vi "MessageHandlerProcess.vi"(10 "InitString":string, 11 "EVE reference in":refnum<data-value>) -> ()   [LabVIEW 2013]
uses:
  001 - MAIN/Class/EVE/EVE.lvclass
  Class/MessageHandler.lvclass
  030 - EVENTS/03 - ToMessageHandlerProcess/enumMessageCriticity.ctl
  030 - EVENTS/03 - ToMessageHandlerProcess/ToMessageHandlerEvent.ctl
  Class/Process/Process.lvclass
panel:
  # "Message handler process ...\n\nProcessus détaché destiné à l'archivage des messages ..."
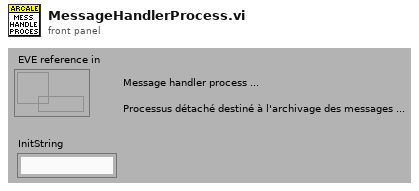
[diagram p1: front panel]
types:
  T1 = typedef "ToMessageHandlerEvent.ctl" = cluster{"date / time":timestamp, "Criticity":T2, "Emitter":string, "Message":string}
  T2 = typedef "enumMessageCriticity.ctl" = enum16{"No error", "Info", "Warning", "Error", "Fatal error"}
  T3 = enum32{"Invalid", "Standard", "Closed", "Hidden", "Minimized", "Maximized"}
  T4 = typedef "EnumToAllProcessesCommand.ctl" = enum16{"Stop all processes", "Autotest"}
  T5 = typedef "ToProcess_EnumCommand.ctl" = enum16{"Show front panel", "Hide front panel"}
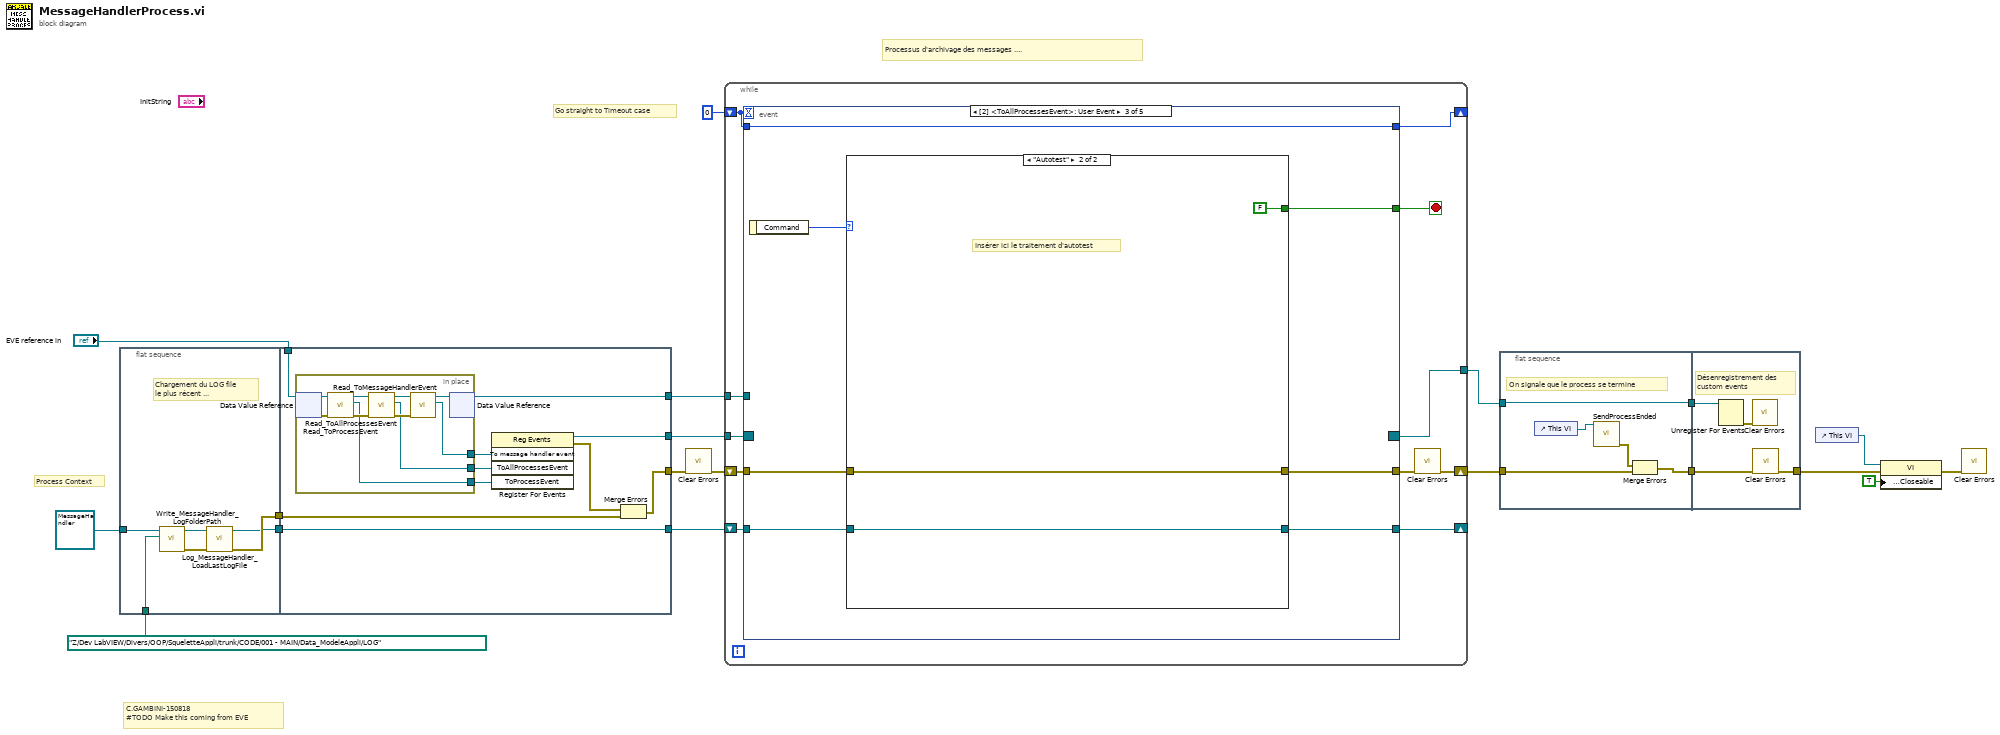
[diagram p0: block diagram]
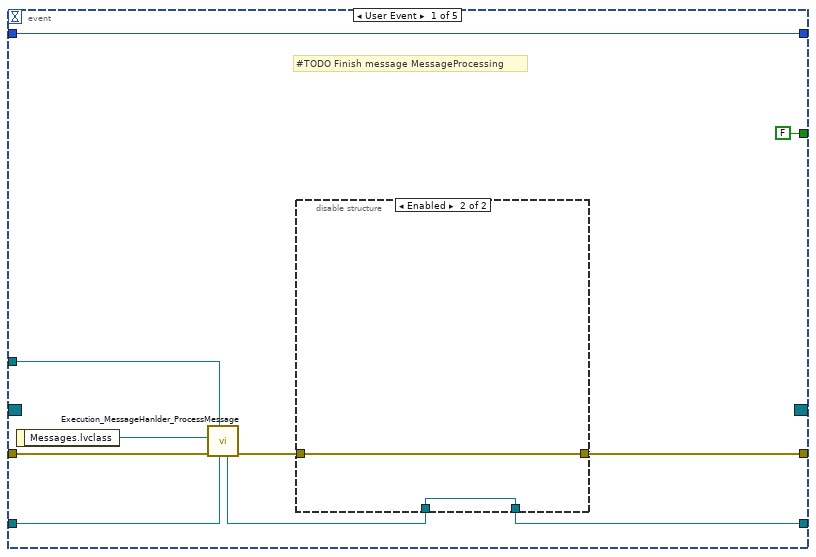
[diagram p2: hidden frame]
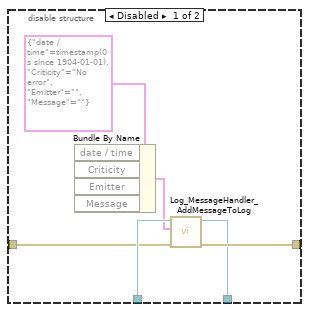
[diagram p3: hidden frame]
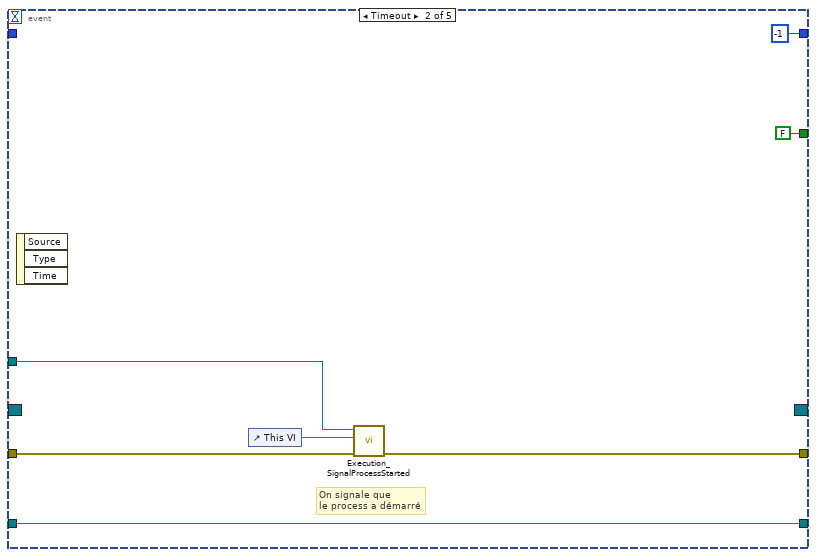
[diagram p4: hidden frame]
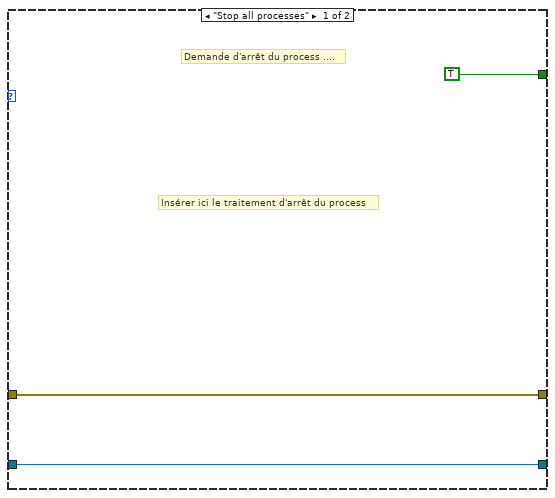
[diagram p5: hidden frame]
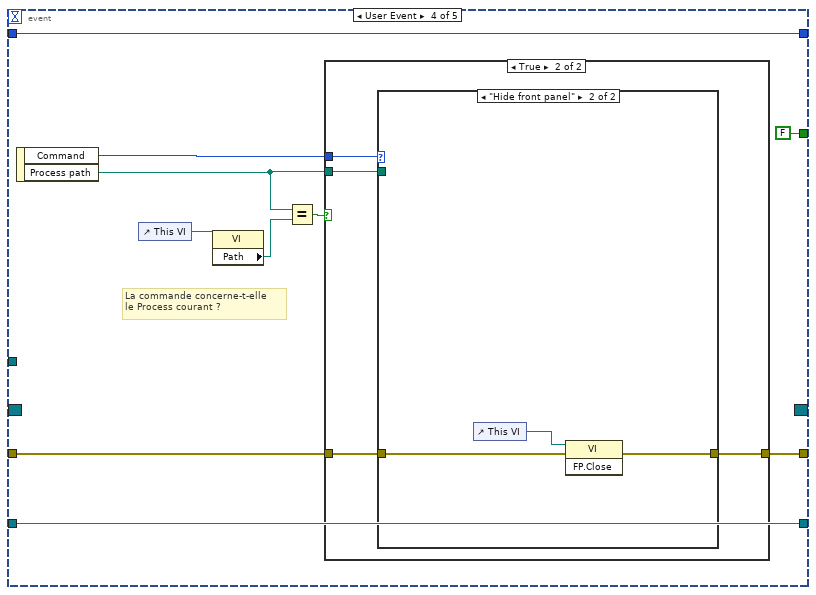
[diagram p6: hidden frame]
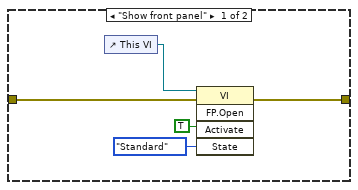
[diagram p8: hidden frame]
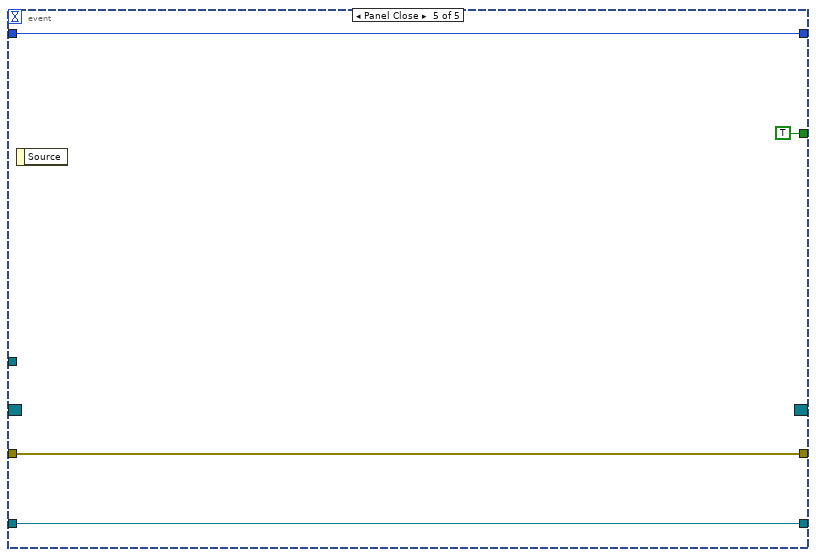
[diagram p9: hidden frame]
diagram:
  # "C.GAMBINI-150818\n#TODO Make this coming from EVE"
  # "Go straight to Timeout case"
  # "Process Context"
  # "Processus d'archivage des messages ...."
  n1 = flat-sequence {
    tunnel: [w22] -> w14
    tunnel: refnum<class "MessageHandler.lvclass"> refnum ("MessageHandler.lvclass") -> [w25]
    tunnel: [w20] -> w13
    tunnel: path "Z:/Dev LabVIEW/Divers/OOP/SqueletteAppli/trunk/CODE/001 - MAIN/Data_ModeleAppli/LOG" -> [w24]
    tunnel: [w34] -> w19
    tunnel: [w32] -> w18
    tunnel: [w33] -> w15
    tunnel: w13 -> [w33]
    tunnel: w14 -> [w35]
    tunnel: "EVE reference in" -> [w30]
    tunnel: [w29] -> w3
    frame #0 {
      # "Chargement du LOG file\nle plus récent ..."
      n2 = call-dynamic "Write_MessageHandler_LogFolderPath.vi"("Log Folder Path"=w24, "MessageHandler in"=w25) -> ("error out"=w23:errorcluster, "MessageHandler out"=w21:refnum<class "MessageHandler.lvclass">)  [unwired: 8 in]
      n3 = call-dynamic "Log_MessageHandler_LoadLastLogFile.vi"("error in"=w23, "MessageHandler in"=w21) -> ("error out"=w22:errorcluster, "MessageHandler out"=w20:refnum<class "MessageHandler.lvclass">)  [unwired: 8 in]
    }
    frame #1 {
      n4 = in-place {
        in-place-border: [w38] -> w28
        in-place-border: [w37] -> w27
        in-place-border: [w36] -> w26
        n5 = in-place-dvr #1(w30) -> (w45:refnum<class "EVE.lvclass">, w44:errorcluster)
        n6 = call-dynamic "Read_ToProcessEvent.vi"("error in (no error)"=w44, "EVE in"=w45) -> ("error out"=w42:errorcluster, "ToProcessEvent"=w36:refnum<user-event>, "EVE out"=w43:refnum<class "EVE.lvclass">)  [unwired: 7 in]
        n7 = call-dynamic "Read_ToAllProcessesEvent.vi"("error in (no error)"=w42, "EVE in"=w43) -> ("error out"=w39:errorcluster, "ToAllProcessesEvent"=w37:refnum<user-event>, "EVE out"=w41:refnum<class "EVE.lvclass">)  [unwired: 7 in]
        n8 = call-dynamic "Read_ToMessageHandlerEvent.vi"("error in (no error)"=w39, "EVE in"=w41) -> ("To message handler event"=w38:refnum<user-event>, "EVE out"=w40:refnum<class "EVE.lvclass">)  [unwired: 7 in, 1 out]
        n9 = in-place-dvr #1(w40) -> (w29:refnum<data-value>)  [unwired: 1 out]
      }
      n10 = register-events(w28, w27, w26) -> (reference out=w32:refnum<event-registration>, error out=w31:errorcluster)  [unwired: 2 in]
      n11 = Merge Errors(w31, w35) -> (w34:errorcluster)
    }
  }
  n12 = call <vilib>:"Clear Errors.vi"("error in (no error)"=w19) -> ("error out"=w12:errorcluster)  [unwired: 6 in]
  n13 = while {
    shift-right: [w52] -> w16
    shift-left: w12 -> [w49]
    tunnel: w18 -> [w55]
    tunnel: [w54] -> w17
    shift-right: [w50] -> _
    shift-left: w15 -> [w51]
    shift-right: [w48] -> _
    shift-left: 0 -> [w47]
    tunnel: w3 -> [w46]
    stop <- w53 stop-if-true
    n14 = event shown="[2] <ToAllProcessesEvent>: User Event" {
      selector: w55 -> [_ _ _ _ _]
      dyn-events: [_ _ _ _ _] -> w54
      timeout: w47 -> [_ _ _ _ _]
      tunnel: w49 -> [w62 w80 w86 w99 w121]
      tunnel: [w66 w79 w85 w98 w121] -> w56
      tunnel: [FALSE FALSE w87 FALSE TRUE] -> w53
      tunnel: w51 -> [w58 w78 w84 w97 w120]
      tunnel: [w65 w78 w83 w97 w120] -> w50
      tunnel: [w60 -1 w82 w95 w118] -> w48
      tunnel: w47 -> [w60 _ w82 w95 w118]
      tunnel: w46 -> [w59 w75 _ _ _]
      event User Event {
        # "#TODO Finish message MessageProcessing"
        n15 = event-data() -> ("Messages.lvclass"=w63:refnum<class "Messages.lvclass">)  [unwired: 1 in]
        n16 = call "Execution_MessageHanlder_ProcessMessage.vi"("MessageHandler.lvclass in"=w58, "EVE reference in"=w59, "error in (no error)"=w62, "Messages.lvclass"=w63) -> ("error out"=w61:errorcluster, "MessageHandler.lvclass out"=w57:refnum<class "MessageHandler.lvclass">)  [unwired: 6 in]
        n17 = disable-structure shown="Enabled" {
          disable-tunnel: [w71 w74] -> w66
          disable-tunnel: w57 -> [w70 w73]
          disable-tunnel: [w69 w73] -> w65
          disable-tunnel: w61 -> [w67 w74]
          frame Disabled {
            n18 = Bundle By Name(cluster=T1 {"date / time"=timestamp(0 s since 1904-01-01), "Criticity"=enum."No error", "Emitter"="", "Message"=""} ("To message handler event")) -> (w68:T1)  [unwired: 4 in]
            n19 = call "Log_MessageHandler_AddMessageToLog.vi"("error in (no error)"=w67, "Messages.lvclass"=w68, "MessageHandler.lvclass in"=w70) -> ("error out"=w71:errorcluster, "MessageHandler.lvclass out"=w69:refnum<class "MessageHandler.lvclass">)  [unwired: 7 in]
          }
          frame Enabled {
          }
        }
      }
      event Timeout {
        # "On signale que\nle process a démarré"
        n20 = event-data() -> ()  [unwired: 1 in, 3 out]
        n21 = control-ref of="This VI"() -> (w76:refnum<vi>)
        n22 = call "Execution_SignalProcessStarted.vi"("error in"=w80, "This VI"=w76, "EVE reference in"=w75) -> ("error out"=w79:errorcluster)  [unwired: 8 in]
      }
      event User Event {
        n23 = event-data() -> ("Command"=w88:T4)  [unwired: 1 in]
        n24 = case shown="\"Autotest\"" w88 {
          tunnel: [TRUE FALSE] -> w87
          tunnel: w86 -> [w90 w94]
          tunnel: [w90 w94] -> w85
          tunnel: w84 -> [w89 w93]
          tunnel: [w89 w93] -> w83
          frame "Stop all processes" {
            # "Insérer ici le traitement d'arrêt du process"
            # "Demande d'arrêt du process ...."
          }
          frame "Autotest" {
            # "Insérer ici le traitement d'autotest"
          }
        }
      }
      event User Event {
        # "La commande concerne-t-elle\nle Process courant ?"
        n25 = event-data() -> ("Command"=w101:T5, "Process path"=w100:path)  [unwired: 1 in]
        n26 = control-ref of="This VI"() -> (w102:refnum<vi>)
        n27 = property class="VI"(reference=w102) -> ("Path"=w103:path)  [unwired: 1 in, 2 out]
        n28 = Equal?(x=w100, y=w103) -> (x = y?=w104:bool)
        n29 = case shown="True" w104 {
          tunnel: w101 -> [_ w109]
          tunnel: w99 -> [w105 w108]
          tunnel: w100 -> [_ w107]
          tunnel: [w105 w106] -> w98
          frame False {
            # "La commande n'est pas pour ce process !"
          }
          frame True {
            n30 = case shown="\"Hide front panel\"" w109 {
              tunnel: w108 -> [w113 w116]
              tunnel: w107 -> [_ _]
              tunnel: [w112 w115] -> w106
              frame "Show front panel" {
                n31 = control-ref of="This VI"() -> (w114:refnum<vi>)
                n32 = invoke class="VI" method="FP.Open"(reference=w114, error in=w113, "Activate"=TRUE ("Activate?"), "State"=T3."Standard") -> (error out=w112:errorcluster)  [unwired: 1 in, 4 out]
              }
              frame "Hide front panel" {
                n33 = control-ref of="This VI"() -> (w117:refnum<vi>)
                n34 = invoke class="VI" method="FP.Close"(reference=w117, error in=w116) -> (error out=w115:errorcluster)  [unwired: 1 in, 2 out]
              }
            }
          }
        }
      }
      event Panel Close {
        n35 = event-data() -> ()  [unwired: 1 in, 1 out]
      }
    }
    n36 = call <vilib>:"Clear Errors.vi"("error in (no error)"=w56) -> ("error out"=w52:errorcluster)  [unwired: 6 in]
  }
  n37 = flat-sequence {
    tunnel: w16 -> [w124]
    tunnel: w17 -> [w126]
    tunnel: [w126] -> w7
    tunnel: [w123] -> w6
    tunnel: [w127] -> w11
    tunnel: w7 -> [w130]
    tunnel: w6 -> [w128]
    frame #0 {
      # "On signale que le process se termine"
      n38 = control-ref of="This VI"() -> (w122:refnum<vi>)
      n39 = call "SendProcessEnded.vi"("Process Refnum"=w122) -> ("error out"=w125:errorcluster)  [unwired: 10 in]
      n40 = Merge Errors(w125, w124) -> (w123:errorcluster)
    }
    frame #1 {
      # "Désenregistrement des\ncustom events"
      n41 = Unregister For Events(event registration refnum=w130) -> (error out=w129:errorcluster)  [unwired: 1 in]
      n42 = call <vilib>:"Clear Errors.vi"("error in (no error)"=w129) -> ()  [unwired: 6 in, 1 out]
      n43 = call <vilib>:"Clear Errors.vi"("error in (no error)"=w128) -> ("error out"=w127:errorcluster)  [unwired: 6 in]
    }
  }
  n44 = control-ref of="This VI"() -> (w10:refnum<vi>)
  n45 = property class="VI"(reference=w10, error in=w11, "Front Panel.Closeable"=TRUE ("Front Panel Window:Closeable")) -> (error out=w8:errorcluster)  [unwired: 1 out]
  n46 = call <vilib>:"Clear Errors.vi"("error in (no error)"=w8) -> ()  [unwired: 6 in, 1 out]
